vi "esp.vi"() -> ()   [LabVIEW 2026]
uses:
  <vilib>/httpClient/LabVIEWHTTPClient.lvlib
panel:
  out "unit":string
  out "value":i32
  out "device_id":string
  in  "stop":bool
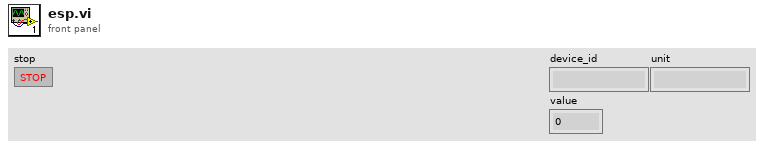
[diagram p1: front panel]
types:
  T1 = cluster{"device_id":string, "value":i32, "unit":string, "timestamp":i32}
  T2 = typedef "LabVIEWHTTPClient.lvlib/ClientHandle.ctl" = refnum<k1>
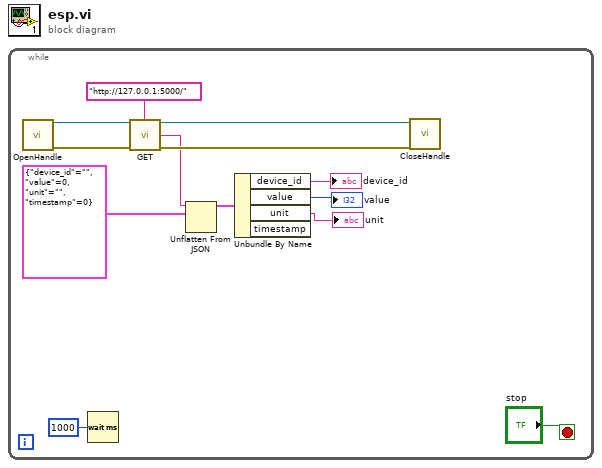
[diagram p0: block diagram]
diagram:
  n1 = while {
    stop <- "stop" stop-if-true
    n2 = call <vilib>:"OpenHandle.vi"() -> ("client handle out"=w13:T2, "error out"=w12:errorcluster)  [unwired: 14 in]
    n3 = Wait (ms)(milliseconds to wait=u32 1000) -> ()  [unwired: 1 out]
    n4 = call <vilib>:"GET.vi"("client handle"=w13, "url"="http://127.0.0.1:5000/", "error in (no error)"=w12) -> ("client handle out"=w11:T2, "body"=w6:string, "error out"=w10:errorcluster)  [unwired: 9 in, 1 out]
    n5 = Unflatten From JSON(JSON string=w6, type and defaults=T1 {"device_id"="", "value"=0, "unit"="", "timestamp"=0}) -> (value=w5:T1)  [unwired: 5 in, 1 out]
    n6 = Unbundle By Name(w5) -> ("device_id"=→"device_id":string, "value"=→"value":i32, "unit"=→"unit":string)  [unwired: 1 out]
    n7 = call <vilib>:"CloseHandle.vi"("client handle"=w11, "error in (no error)"=w10) -> ()  [unwired: 13 in, 1 out]
  }
